vi "btnController.vi"(7 "state":enum16{"Init", "enable"}(ring), 8 "error in (no error)":errorcluster caption="에러 입력(에러 없음)", 10 "2dArray":string[][](table), 11 "btnGroup":refnum<vi>) -> (0 "error out":errorcluster caption="에러 출력")   [LabVIEW 2019]
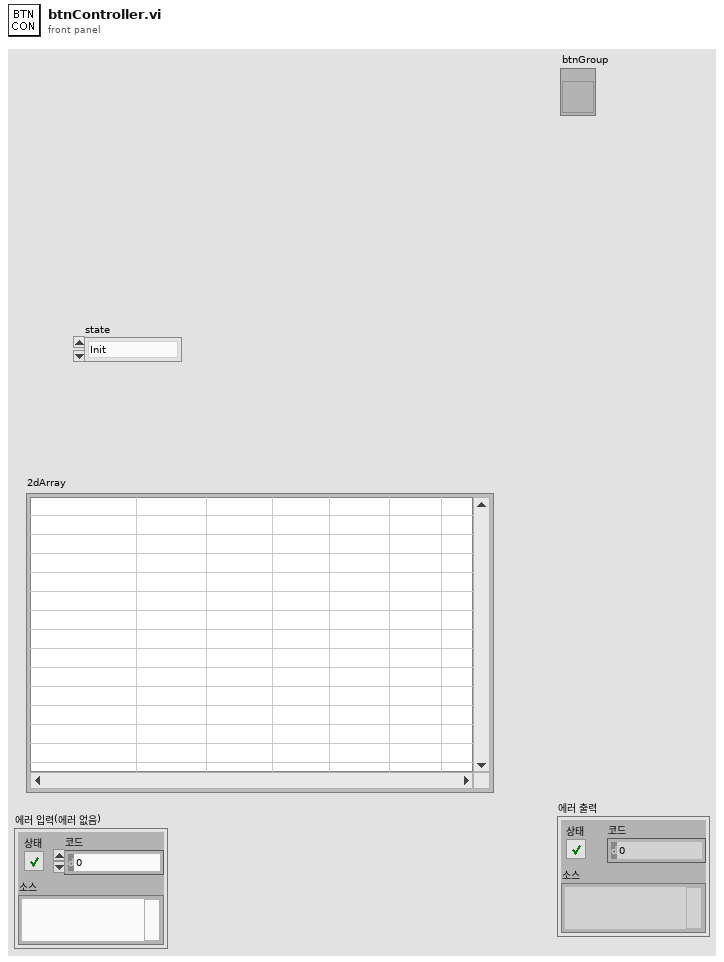
[diagram p1: front panel]
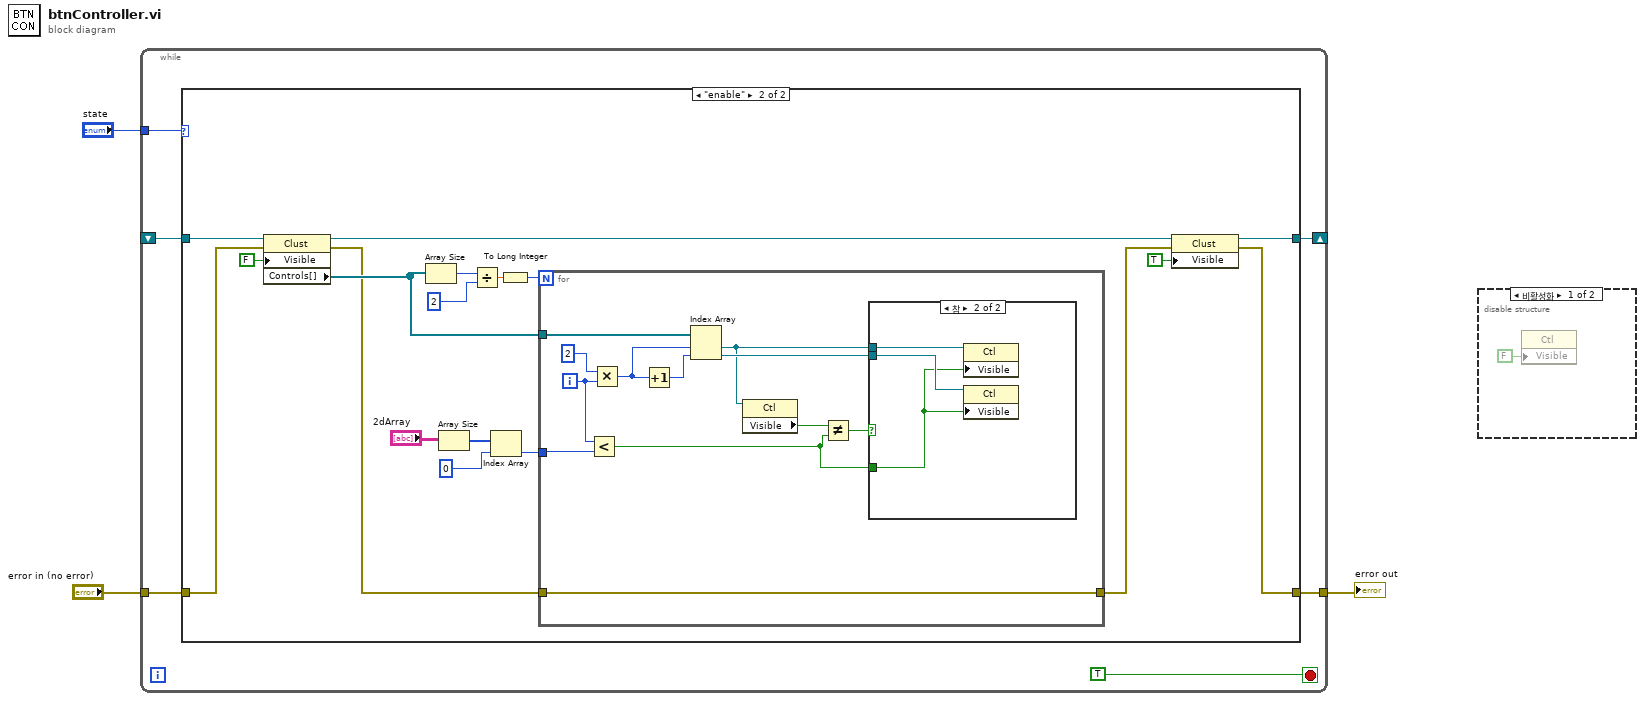
[diagram p0: block diagram]
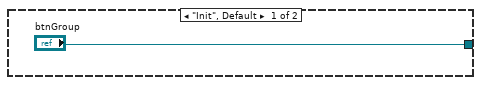
[diagram p3: hidden frame]
diagram:
  n1 = while {
    tunnel: "state" -> [w9]
    shift-right: [w8] -> _
    shift-left: _ -> [w7]
    tunnel: "error in (no error)" -> [w5]
    tunnel: [w4] -> w1
    stop <- TRUE stop-if-true
    n2 = case shown="\"enable\"" w9 {
      tunnel: ["btnGroup" w14] -> w8
      tunnel: w7 -> [_ w15]
      tunnel: w5 -> [_ w16]
      tunnel: [_ w12] -> w4
      frame "Init", Default {
      }
      frame "enable" {
        n3 = property class="Clust"(reference=w15, error in=w16, "Visible"=FALSE ("보이기")) -> (error out=w17:errorcluster, "Controls[]"=w19:refnum<vi>[])  [unwired: 1 out]
        n4 = Array Size(array=w19) -> (size(s)=w27:i32)
        n5 = Array Size(array="2dArray") -> (size(s)=w22:i32[])
        n6 = Divide(x=w27, y=2) -> (x/y=w26:dbl)
        n7 = Index Array(array=w22, index=0 ("인덱스")) -> (element=w20:i32)
        n8 = To Long Integer(number=w26) -> (32bit integer=w24:i32)
        n9 = for {
          N: w24 -> [_]
          tunnel: w20 -> [w34]
          tunnel: w19 -> [w29]
          tunnel: w17 -> [w28]
          tunnel: [w28] -> w13
          i -> [w35]
          n10 = Less?(x=w35, y=w34) -> (x < y?=w30:bool)
          n11 = Multiply(x=2, y=w35) -> (x*y=w37:i32)
          n12 = Increment(x=w37) -> (x+1=w38:i32)
          n13 = Index Array(array=w29, index #1=w37, index #2=w38) -> (element #1=w33:refnum<vi>, element #2=w36:refnum<vi>)
          n14 = property class="Ctl"(reference=w33) -> ("Visible"=w32:bool)  [unwired: 1 in, 2 out]
          n15 = Not Equal?(x=w32, y=w30) -> (x != y?=w31:bool)
          n16 = case shown="참" w31 {
            tunnel: w36 -> [_ w42]
            tunnel: w33 -> [_ w41]
            tunnel: w30 -> [_ w40]
            frame False {
            }
            frame True {
              n17 = property class="Ctl"(reference=w41, "Visible"=w40) -> ()  [unwired: 1 in, 2 out]
              n18 = property class="Ctl"(reference=w42, "Visible"=w40) -> ()  [unwired: 1 in, 2 out]
            }
          }
        }
        n19 = property class="Clust"(reference=w15, error in=w13, "Visible"=TRUE ("보이기")) -> (reference out=w14:refnum<vi>, error out=w12:errorcluster)
      }
    }
  }
  "error out" <- w1
  n20 = disable-structure shown="비활성화" {
    frame Disabled {
      n21 = property class="Ctl"("Visible"=FALSE ("보이기")) -> ()  [unwired: 2 in, 2 out]
    }
    frame Enabled {
    }
  }
